vi "Stop Core.vi"(10 "final error code":i32, 11 "Process Model in":refnum<class "Process Model.lvclass">) -> (3 "Process Model out":refnum<class "Process Model.lvclass">)   [LabVIEW 2017, in "Process Model.lvlib" / "Process Model.lvclass"]
doc: "(<B>Filename</B>: Actor Framework.lvlib:Actor.lvclass:Stop Core.vi)\n\nDefines what the actor does before it stops. Use the <B>final error code</B> input to determine whether the actor shut down in response to an error.\n\nBy default, this method does nothing. A descendant class may override it to define behavior, such as shutting down any processes the actor initiated in its override of the Actor Core method."
uses:
  <vilib>/gpm_packages/@cs/Car wash/Process Model/Process Model/Process Model.lvclass
  <vilib>/gpm_packages/@cs/test-executive/Source/Test Executive/TestExecutive Ref/TestExecutive Ref.lvclass
  <vilib>/gpm_packages/@cs/Car wash/iProcess Model/iProcess Model/iProcess Model.lvclass
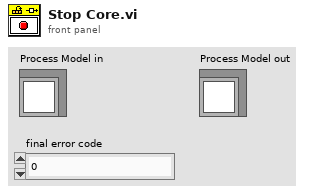
[diagram p1: front panel]
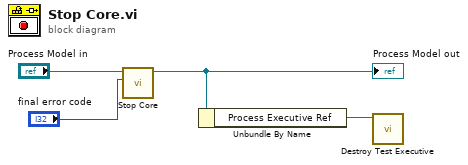
[diagram p0: block diagram]
diagram:
  n1 = call-parent "Stop Core.vi"("final error code"="final error code", "IObserver in"="Process Model in") -> ("IObserver out"=w2:refnum<class "Process Model.lvclass">)  [unwired: 9 in]
  "Process Model out" <- w2
  n2 = Unbundle By Name(w2) -> ("Process Executive Ref"=w1:refnum<data-value>)
  n3 = call <vilib>:"Destroy Test Executive.vi"("Test Executive Ref"=w1) -> ()  [unwired: 10 in, 1 out]
